vi "multi-mode-acquisition.vi"() -> ()   [LabVIEW 2014]
doc: "Acquires sequences from the Andor iXon camera. \"Multi-mode\" means that the VI can be configured to sequentially acquire frames in multiple modes with different light sources and numbers of frames in each mode. Each mode is collected into a separate aquisition directory. Acquisition can be time-lapsed with a settable delay interval between cycles; the selected laser(s) are shuttered whilst not acquiring. The ixon setup acquisition.vi front panel is displayed so that the user can set the acquisition parameters before acquiring."
uses:
  SubVIs/ctt's/Image size and binning.ctl
  SubVIs/ctt's/Camera Setup Acquisition.ctl
  SubVIs/ctt's/acquisition protocol multimode.ctl
  Shutter Control/Shutter SubVIs/ctts/laser shutters.ctl
  SubVIs/ctt's/Video acquisition state1.ctl
  <vilib>/vision/Image Controls.llb/IMAQ Image.ctl
  Shutter Control/Shutter SubVIs/ctts/user event shutter global.ctl
  SubVIs/Globals/Initilize Globals.vi
  File Directory/File-Locations-Global.vi
  TIRF Lock/autofocus-globals.vi
  Stage Control/stage-controller-globals.vi
panel:
  in  "Exposure Time (sec)":sgl(slide)=0.1 scale=0.001..10.0 scale format="%#_1g"
  in  "EM CCD Gain":u16(slide)=300 scale=0.01..300.0
  in  "Acquisition directory root path":path=path "c:/scratch"
  in  "Max Cycles":i32
  in  "Cycle Interval (s)":dbl format="%_2g"
  in  "Scan Fields":bool
  in  "Scan Field Options":T1(radio)
  in  "Max. number of acquisition files":i8(slide)=10 scale=0.0..50.0
  in  "Acquisition Protocol":T2
  in  "Quit":bool
  in  "Start":bool
  in  "Acquisition Parameters":T4={"Set Acquisition Mode"=enum."Single Scan", "Trigger Mode"=enum."Internal", "Set VS Speed"=1.0, "Pixel Rate"=enum."Standard CCD 3 Mhz 14 bits", "V Shift Amplitude"=enum."+1", "Readout Mode"=enum."Image", "Single Track \nSettings"={"centre"=0, "height"=1}, "Preamp Gain"=enum."1.0", "Number of\nAccumulations"=0, "Number of Kinetics"=1, "Accumulation\nCycle (s)"=1.0, "Kinetic Cycle Time (s)"=1.0, "High Capacity?"=FALSE} {"Single Track \nSettings"."centre" min=0 max=1024; "Single Track \nSettings"."height" min=1 max=1024; "Set VS Speed" min=0.0 format="%#_2f"}
  in  "Image Size":T5={"H Bin"=1.0, "V Bin"=1.0, "Left"=1.0, "Right"=1024.0, "Top"=1.0, "Bottom"=1024.0} {"V Bin" min=0.0; "H Bin" min=0.0 step=1.0}
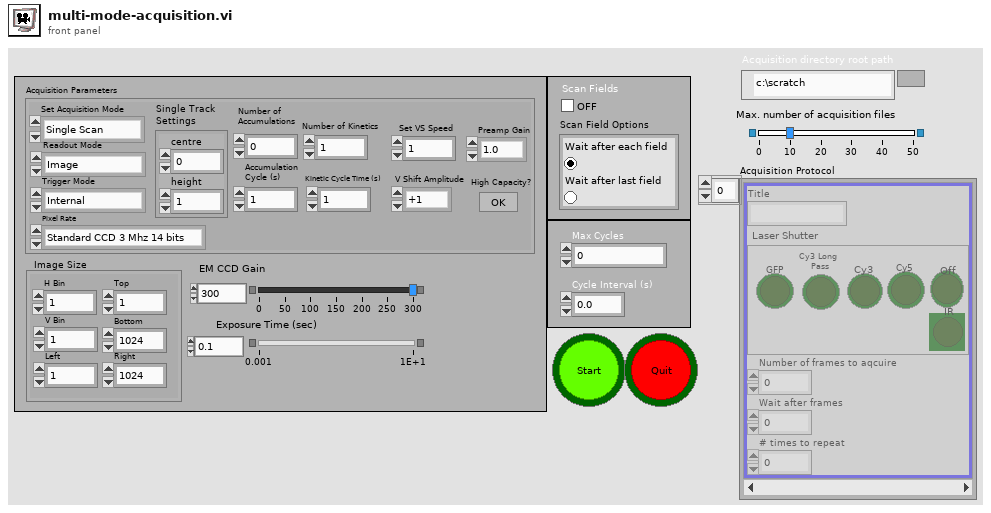
[diagram p1: front panel]
types:
  T1 = enum32{"Wait after each field", "Wait after last field"}
  T2 = typedef "acquisition protocol multimode.ctl" = cluster{"Title":string, "Laser Shutter":T3, "Number of frames to aqcuire":dbl, "Wait after frames":dbl, "# times to repeat":u32}[]
  T3 = typedef "laser shutters.ctl" = enum32{"No Selection", "GFP", "Cy3 Long \nPass", "Cy3", "Cy5", "Off", "IR"}
  T4 = typedef "Camera Setup Acquisition.ctl" = cluster{"Set Acquisition Mode":enum16{"(do nothing)", "Single Scan", "Accumulate", "Kinetics", "Fast Kinetics", "Run till abort"}, "Trigger Mode":enum16{"Internal", "External"}, "Set VS Speed":dbl, "Pixel Rate":enum16{"EM CCD 10 Mhz 14 bits", "EM CCD 5 Mhz 14 bits", "EM CCD 3 Mhz 14 bits", "EM CCD 1 Mhz 16 bits", "Standard CCD 3 Mhz 14 bits", "Standard CCD 1 Mhz 16 bits"}, "V Shift Amplitude":enum16{"normal", "+1", "+2", "+3", "+4"}, "Readout Mode":enum16{"Full Vertical Binning", "Multi-Track", "Random-Track", "Single-Track", "Image"}, "Single Track \nSettings":cluster{"centre":i32, "height":i32}, "Preamp Gain":enum16{"1.0", "2.4", "5.0"}, "Number of\nAccumulations":i32, "Number of Kinetics":i32, "Accumulation\nCycle (s)":dbl, "Kinetic Cycle Time (s)":dbl, "High Capacity?":bool}
  T5 = typedef "Image size and binning.ctl" = cluster{"H Bin":dbl, "V Bin":dbl, "Left":dbl, "Right":dbl, "Top":dbl, "Bottom":dbl}
  T6 = typedef "user event shutter global.ctl" = cluster{"Camera Shutter":bool, "Laser Shutter":enum32{"No Selection", "GFP", "Cy3 Long \nPass", "Cy3", "Cy5", "Off", "IR"}}
  T7 = enum32{"None", "Manual", "Auto - Image analysis", "Auto - Retro-reflection"}
  T8 = enum32{"No Selection", "GFP", "Cy3 Long \nPass", "Cy3", "Cy5", "Off", "IR"}
  T9 = cluster{"Title":string, "Laser Shutter":T3, "Number of frames to aqcuire":dbl, "Wait after frames":dbl, "# times to repeat":u32}
  T10 = cluster{"H Bin":dbl, "V Bin":dbl, "Left":dbl, "Right":dbl, "Top":dbl, "Bottom":dbl}
  T11 = cluster{"Frame Size (bytes)":i32, "Max Time (min)":i32, "Max Frames":i32, "Frames per acquisition file":i32, "Max time (s)":i32, "Max Space Req'd. (Gb)":dbl}
  T12 = typedef "Video acquisition state1.ctl" = cluster{"Pixel depth":enum32{"8 bits", "16 bits", "Float", "Complex", "RGB Chunky", "Compressed"}, "Width":dbl, "Height":dbl, "Buffer":T13, "Frames Acquired":u32, "Time of 1st frame":dbl, "TTB element zero":u32, "File Offsets Array":cluster{"offset":i32, "file number":u8}[], "TTB Array":u32[], "Sum Image (for averaging)":T13, "Time at end of last acquisition (ms)":u32, "Flow rate array":dbl[], "Temperature array":dbl[], "Field array":u16[], "Stage xyz array":dbl[][], "Current Filter Wheel Array":string[], "Laser Shutter Array":enum32{"No Selection", "GFP", "Cy3 Long \nPass", "Cy3", "Cy5", "Off", "IR"}[]}
  T13 = typedef "IMAQ Image.ctl" = refnum<image>
  T14 = typedef "Sequence file handle.ctl" = cluster{"Sequence files directory path":path, "Sequence files refnum array":refnum<file>[]}
  T15 = cluster{"Sequence files directory path":path, "Sequence files refnum array":refnum<file>[]}
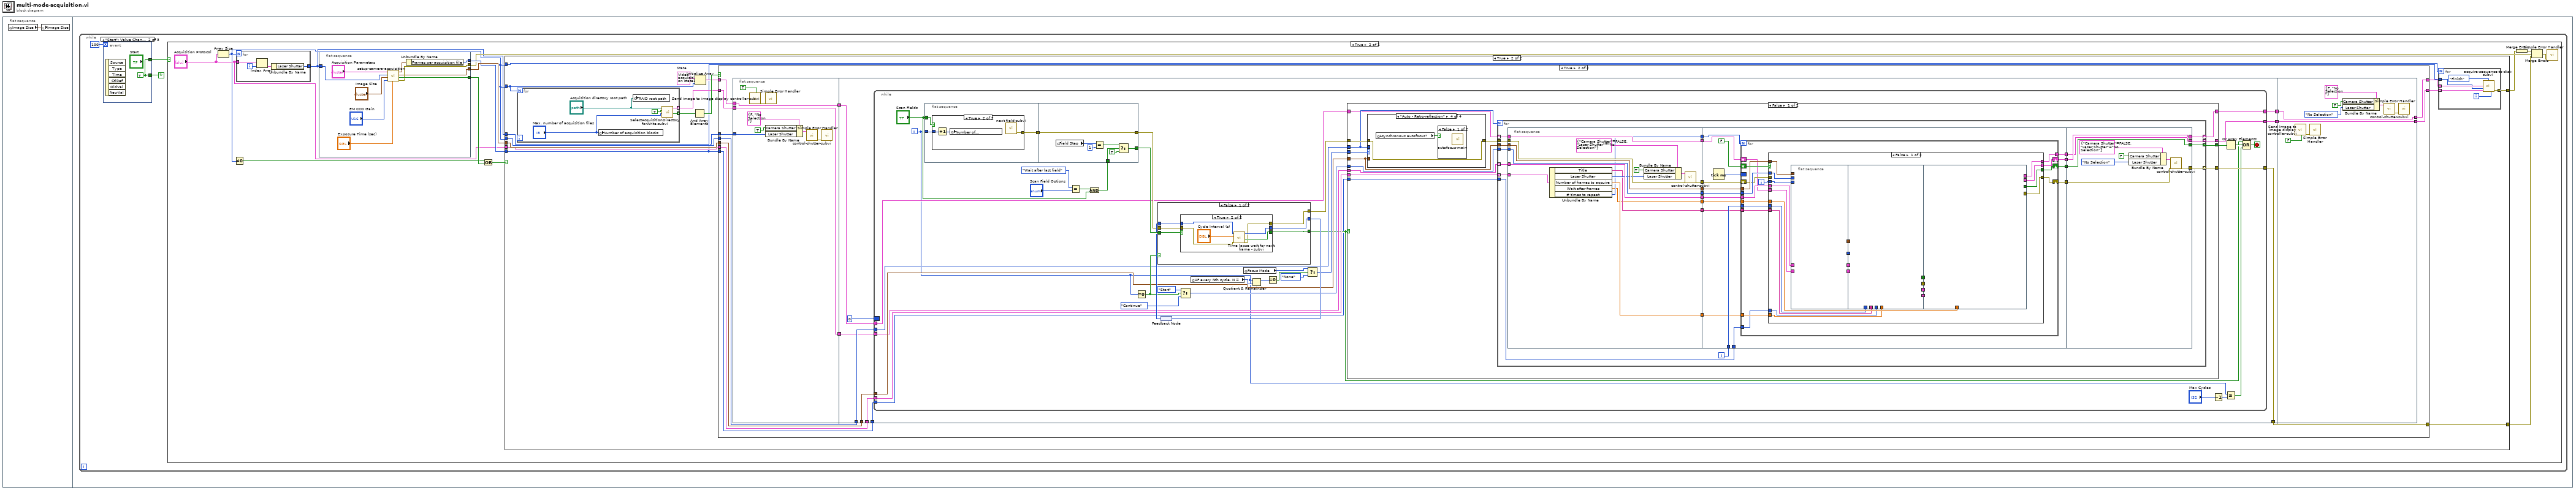
[diagram p0: block diagram]
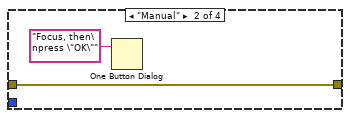
[diagram p7: hidden frame]
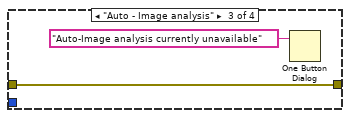
[diagram p8: hidden frame]
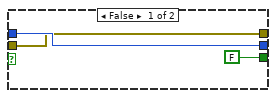
[diagram p11: hidden frame]
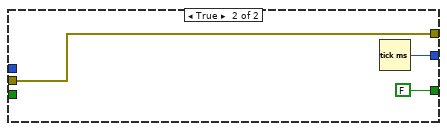
[diagram p12: hidden frame]
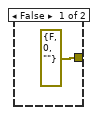
[diagram p13: hidden frame]
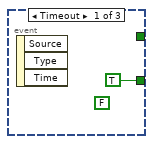
[diagram p14: hidden frame]
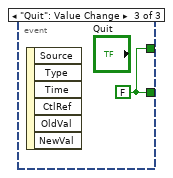
[diagram p15: hidden frame]
diagram:
  n1 = flat-sequence {
    frame #0 {
      n2 = global read "Initilize Globals.vi" "Image Size"() -> (w1:T5)
      n3 = local write "Image Size"(w1) -> ()
    }
    frame #1 {
      n4 = while {
        stop <- w3 continue-if-true
        n5 = event shown="[1] \"Start\": Value Change" {
          selector: _ -> [_ _ _]
          dyn-events: _ -> [_ _ _]
          timeout: 100 -> [_ _ _]
          tunnel: [TRUE w337 w338] -> w3
          tunnel: [_ w337 w338] -> w2
          event Timeout {
            (unwired) FALSE
            n6 = event-data() -> ()  [unwired: 1 in, 3 out]
          }
          event "Start": Value Change {
            w337 = TRUE
            n7 = event-data() -> ()  [unwired: 1 in, 6 out]
          }
          event "Quit": Value Change {
            w338 = FALSE
            n8 = event-data() -> ()  [unwired: 1 in, 6 out]
          }
        }
        n9 = case shown="True" w2 {
          frame False {
          }
          frame True {
            n10 = Array Size(array="Acquisition Protocol") -> (size(s)=w9:i32)
            n11 = Not Equal To 0?(x=w9) -> (x != 0?=w5:bool)
            n12 = for {
              N: w9 -> [_]
              tunnel: "Acquisition Protocol" -> [w21]
              tunnel: [w18] -> w6
              i -> [w20]
              n13 = Index Array(array=w21, index=w20) -> (element=w19:T9)
              n14 = Unbundle By Name(w19) -> ("Laser Shutter"=w18:T3)
            }
            n15 = flat-sequence {
              tunnel: [w331] -> w16
              tunnel: [w330] -> w11
              tunnel: [w328] -> w15
              tunnel: [w335] -> w12
              tunnel: w6 -> [w332]
              frame #0 {
                n16 = call "setup-camera-acquisition.vi"("Exposure Time (sec)"="Exposure Time (sec)", "EM CCD Gain"="EM CCD Gain", "Image Size"="Image Size", "Laser Shutter"=w332, "Acquisition Parameters"="Acquisition Parameters") -> ("Error Out"=w330:errorcluster, "Continue with \nacquisition?"=w331:bool, "Image Size Out"=w328:T10, "File properties"=w329:T11)  [unwired: 3 in]
                n17 = Unbundle By Name(w329) -> ("Frames per acquisition file"=w335:i32)
              }
            }
            n18 = Or(x=w5, y=w16) -> (x .or. y?=w17:bool)
            n19 = case shown="True" w17 {
              tunnel: w9 -> [_ w37]
              tunnel: w15 -> [_ w33]
              tunnel: "Acquisition Protocol" -> [_ w32]
              tunnel: w9 -> [_ w31]
              tunnel: [_ w30] -> w14
              tunnel: w9 -> [_ w29]
              tunnel: w12 -> [_ w23]
              tunnel: [_ w26] -> w7
              tunnel: w6 -> [_ w22]
              frame False {
              }
              frame True {
                w36 = T12 {"Pixel depth"=enum."8 bits", "Width"=0.0, "Height"=0.0, "Buffer"=refnum, "Frames Acquired"=0, "Time of 1st frame"=0.0, "TTB element zero"=0, "File Offsets Array"=[], "TTB Array"=[], "Sum Image (for averaging)"=refnum, "Time at end of last acquisition (ms)"=0, "Flow rate array"=[], "Temperature array"=[], "Field array"=[], "Stage xyz array"=[], "Current Filter Wheel Array"=[], "Laser Shutter Array"=[]}  # State
                n20 = for {
                  N: w37 -> [_]
                  tunnel: [w323] -> w35 mode=indexing
                  tunnel: [w322] -> w28 mode=indexing
                  n21 = global write "Initilize Globals.vi" "Number of acquisition blocks"("Max. number of acquisition files") -> ()
                  n22 = global write "File-Locations-Global.vi" "RAID root path"("Acquisition directory root path") -> ()
                  n23 = call "SelectAcquisitionDirectoryforWrite-subvi.vi"("Number of acquisition files"="Max. number of acquisition files", "Autostart?"=TRUE, "Acquisition directory root path"="Acquisition directory root path") -> ("OK?"=w323:bool, "Sequence files handle"=w322:T14)  [unwired: 7 in]
                }
                n24 = And Array Elements(Boolean array=w35) -> (logical AND=w34:bool)
                n25 = Initialize Array(w36, w37) -> (w27:T12[])
                n26 = case shown="True" w34 {
                  tunnel: w33 -> [_ w59]
                  tunnel: w32 -> [_ w58]
                  tunnel: w31 -> [_ w57]
                  tunnel: [_ w56] -> w30
                  tunnel: w28 -> [w45 w54]
                  tunnel: w27 -> [w44 w48]
                  tunnel: w23 -> [_ w53]
                  tunnel: [w44 w51] -> w25
                  tunnel: [w45 w49] -> w24
                  tunnel: w22 -> [_ w46]
                  frame False {
                  }
                  frame True {
                    n27 = flat-sequence {
                      tunnel: [w62] -> w55
                      tunnel: w54 -> [w62]
                      tunnel: w48 -> [w61]
                      tunnel: [w61] -> w47
                      tunnel: w46 -> [w60]
                      tunnel: w59 -> [w77]
                      tunnel: w58 -> [w76]
                      tunnel: w57 -> [w75]
                      tunnel: [w74] -> w56
                      tunnel: w55 -> [w73]
                      tunnel: w53 -> [w72]
                      tunnel: [w71] -> w52
                      tunnel: [w70] -> w50
                      tunnel: w47 -> [w69]
                      tunnel: w52 -> [w313]
                      tunnel: [w313] -> w51
                      tunnel: w50 -> [w312]
                      tunnel: [w312] -> w49
                      frame #0 {
                        n28 = call "Send image to image display controller-subvi.vi"("Start display controller?"=TRUE) -> ("error out"=w64:errorcluster)  [unwired: 8 in, 1 out]
                        n29 = call <vilib>:"Simple Error Handler.vi"("error in (no error)"=w64) -> ()  [unwired: 1 in, 8 out]
                        n30 = Bundle By Name(cluster=T6 {"Camera Shutter"=FALSE, "Laser Shutter"=enum."No Selection"} ("Shutter Control"), "Camera Shutter"=TRUE, "Laser Shutter"=w60) -> (w66:T6)
                        n31 = call "control-shutter-subvi.vi"("Shutter Control"=w66) -> ("Error Out"=w65:errorcluster)  [unwired: 10 in]
                        n32 = call <vilib>:"Simple Error Handler.vi"("error in (no error)"=w65) -> ()  [unwired: 1 in, 8 out]
                      }
                      frame #1 {
                        n33 = while {
                          border: 0 -> [_]
                          tunnel: w77 -> [w98]
                          tunnel: w76 -> [w95]
                          tunnel: w75 -> [w94]
                          tunnel: [w91] -> w74
                          tunnel: w73 -> [w89]
                          tunnel: w69 -> [w86]
                          tunnel: w72 -> [w85]
                          tunnel: [w84] -> w71
                          tunnel: [w83] -> w70
                          i -> [w79]
                          stop <- w92 stop-if-true
                          n34 = flat-sequence {
                            tunnel: "Scan Fields" -> [w300]
                            tunnel: [w299] -> w112
                            tunnel: w79 -> [w298]
                            tunnel: w113 -> [w310]
                            tunnel: w112 -> [w309]
                            tunnel: [w309] -> w97
                            tunnel: [w308] -> w111
                            frame #0 {
                              n35 = case shown="True" w300 {
                                tunnel: [errorcluster {"status"=FALSE, "code"=0, "source"=""} ("Error Out") w304] -> w299
                                tunnel: w298 -> [_ w303]
                                frame False {
                                }
                                frame True {
                                n36 = Increment(x=w303) -> (x+1=w302:i32)
                                n37 = global write "stage-controller-globals.vi" "Number of \nField Steps"(w302) -> ()
                                n38 = call "next field-subvi.vi"() -> ("Error Out"=w304:errorcluster)  [unwired: 11 in]
                                }
                              }
                            }
                            frame #1 {
                              n39 = global read "stage-controller-globals.vi" "Field Step"() -> (w305:u32)
                              n40 = Equal?(x=w305, y=u32 1) -> (x = y?=w307:bool)
                              n41 = Select(t=w307, s=w310, f=TRUE) -> (s? t:f=w308:bool)
                            }
                          }
                          n42 = Equal?(x=T1."Wait after last field" ("y"), y="Scan Field Options") -> (x = y?=w116:bool)
                          n43 = And(x=w116, y="Scan Fields") -> (x .and. y?=w113:bool)
                          n44 = Equal To 0?(x=w79) -> (x = 0?=w108:bool)
                          n45 = feedback #1() -> (w109:u32)
                          n46 = case shown="False" w108 {
                            tunnel: w111 -> [w285 _]
                            tunnel: [w283 w297] -> w110
                            tunnel: w109 -> [w282 _]
                            tunnel: [w284 FALSE] -> w87
                            tunnel: w97 -> [w281 w295]
                            tunnel: [w280 w295] -> w96
                            frame False {
                              n47 = case shown="True" w285 {
                                tunnel: [FALSE w291] -> w284
                                tunnel: [w287 w293] -> w283
                                tunnel: w282 -> [w287 w294]
                                tunnel: w281 -> [w286 w290]
                                tunnel: [w286 w289] -> w280
                                frame False {
                                }
                                frame True {
                                n48 = call "Time lapse wait for next frame - subvi.vi"("Error In"=w290, "Frame Interval (s)"="Cycle Interval (s)", "Time of last frame in"=w294) -> ("Error Out"=w289:errorcluster, "Stopped?"=w291:bool, "Time of this frame out (ms)"=w293:i32)  [unwired: 5 in, 1 out]
                                }
                              }
                            }
                            frame True {
                              n49 = Tick Count (ms)() -> (millisecond timer value=w297:u32)
                            }
                          }
                          n50 = feedback-in #1(w110) -> ()
                          n51 = Select(t=enum16{"Start", "Continue", "Finish"}."Start" ("Operation"), s=w108, f=enum16{"Start", "Continue", "Finish"}."Continue" ("Operation")) -> (s? t:f=w102:enum16{"Start", "Continue", "Finish"})
                          n52 = global read "autofocus-globals.vi" "AF every Nth cycle, N ="() -> (w105:u32)
                          n53 = global read "autofocus-globals.vi" "Focus Mode"() -> (w103:T7)
                          n54 = Quotient & Remainder(x=w79, y=w105) -> (x-y*floor(x/y)=w107:u32)  [unwired: 1 out]
                          n55 = Equal To 0?(x=w107) -> (x = 0?=w106:bool)
                          n56 = Select(t=w103, s=w106, f=T7."None") -> (s? t:f=w101:T7)
                          n57 = case shown="False" w87 {
                            tunnel: w102 -> [w123 _]
                            tunnel: w101 -> [w130 _]
                            tunnel: w98 -> [w122 _]
                            tunnel: w96 -> [w129 _]
                            tunnel: w95 -> [w128 _]
                            tunnel: w94 -> [w127 _]
                            tunnel: [w126 _] -> w91
                            tunnel: [w125 _] -> w90
                            tunnel: w89 -> [w124 w279]
                            tunnel: w86 -> [w121 w278]
                            tunnel: w85 -> [w120 _]
                            tunnel: [w118 w278] -> w84
                            tunnel: [w117 w279] -> w83
                            frame False {
                              n58 = case shown="\"Auto - Retro-reflection\"" w130 {
                                tunnel: w122 -> [_ _ _ _]
                                tunnel: w129 -> [w271 w272 w275 w276]
                                tunnel: [w271 w272 w275 w276] -> w119
                                tunnel: w127 -> [_ _ _ _]
                                frame "None", Default {
                                }
                                frame "Manual" {
                                n59 = One Button Dialog(message="Focus, then\npress \"OK\"") -> ()  [unwired: 2 out]
                                }
                                frame "Auto - Image analysis" {
                                n60 = One Button Dialog(message="Auto-Image analysis currently unavailable") -> ()  [unwired: 2 out]
                                }
                                frame "Auto - Retro-reflection" {
                                n61 = global read "autofocus-globals.vi" "Asynchronous autofocus?"() -> (w277:bool)
                                n62 = case shown="False" w277 {
                                frame False {
                                n63 = call "autofocus-main.vi"() -> ()  [unwired: 12 in]
                                }
                                frame True {
                                }
                                }
                                }
                              }
                              n64 = for {
                                N: w127 -> [_]
                                tunnel: w128 -> [w140] mode=indexing
                                tunnel: [w131] -> w126 mode=indexing
                                tunnel: [w155] -> w125 mode=indexing
                                tunnel: w124 -> [w154] mode=indexing
                                tunnel: w123 -> [w153]
                                tunnel: w122 -> [w152]
                                tunnel: w121 -> [w146] mode=indexing
                                tunnel: w120 -> [w150]
                                tunnel: w119 -> [w149]
                                tunnel: [w148] -> w118 mode=indexing
                                tunnel: [w147] -> w117 mode=indexing
                                i -> [w151]
                                n65 = flat-sequence {
                                tunnel: w146 -> [w167]
                                tunnel: w149 -> [w165]
                                tunnel: w152 -> [w168]
                                tunnel: w153 -> [w169]
                                tunnel: w154 -> [w170]
                                tunnel: [w170] -> w145
                                tunnel: [w169] -> w144
                                tunnel: [w168] -> w143
                                tunnel: [w164] -> w142
                                tunnel: [w167] -> w141
                                tunnel: w140 -> [w166]
                                tunnel: [w159] -> w139
                                tunnel: [w158] -> w138
                                tunnel: [w157] -> w137
                                tunnel: [w156] -> w136
                                tunnel: w151 -> [w182]
                                tunnel: w150 -> [w181]
                                tunnel: w145 -> [w185]
                                tunnel: w144 -> [w184]
                                tunnel: w143 -> [w183]
                                tunnel: w142 -> [w180]
                                tunnel: w141 -> [w176]
                                tunnel: w139 -> [w175]
                                tunnel: w138 -> [w174]
                                tunnel: w137 -> [w173]
                                tunnel: w136 -> [w172]
                                tunnel: [w187] -> w135
                                tunnel: [w179] -> w134
                                tunnel: [w178] -> w133
                                tunnel: [w171] -> w132
                                tunnel: [w268] -> w147
                                tunnel: [w269] -> w148
                                tunnel: [w270] -> w155
                                tunnel: w135 -> [w270]
                                tunnel: w134 -> [w269]
                                tunnel: w133 -> [w268]
                                tunnel: w132 -> [w267]
                                tunnel: [w266] -> w131
                                frame #0 {
                                n66 = Unbundle By Name(w166) -> ("Title"=w159:string, "Laser Shutter"=w160:T3, "Number of frames to aqcuire"=w158:dbl, "Wait after frames"=w156:dbl, "# times to repeat"=w157:u32)
                                n67 = Bundle By Name(cluster=T6 {"Camera Shutter"=FALSE, "Laser Shutter"=enum."No Selection"} ("Shutter Control"), "Camera Shutter"=TRUE, "Laser Shutter"=w160) -> (w162:T6)
                                n68 = call "control-shutter-subvi.vi"("Error In"=w165, "Shutter Control"=w162) -> ("Error Out"=w164:errorcluster)  [unwired: 9 in]
                                }
                                frame #1 {
                                n69 = Tick Count (ms)() -> (millisecond timer value=w177:u32)
                                n70 = for {
                                N: w173 -> [_]
                                shift-right: [w203] -> w171
                                shift-left: w180 -> [w191]
                                shift-right: [w202] -> w187
                                shift-left: FALSE -> [w201]
                                tunnel: w172 -> [w200]
                                tunnel: w185 -> [w199]
                                tunnel: w175 -> [w198]
                                tunnel: w174 -> [w197]
                                tunnel: w184 -> [w196]
                                tunnel: w183 -> [w195]
                                tunnel: w182 -> [w193]
                                tunnel: w181 -> [w192]
                                tunnel: [w189] -> w178
                                border: w177 -> [_]
                                shift-right: [w190] -> w179
                                shift-left: w176 -> [w188]
                                i -> [w194]
                                n71 = case shown="False" w201 {
                                selector: w201 -> [_ w260]
                                tunnel: [w225 w261] -> w203
                                tunnel: [w224 w260] -> w202
                                tunnel: w200 -> [w223 _]
                                tunnel: w199 -> [w222 w258]
                                tunnel: w198 -> [w220 _]
                                tunnel: w197 -> [w219 _]
                                tunnel: w196 -> [w218 _]
                                tunnel: w195 -> [w217 _]
                                tunnel: w194 -> [w215 _]
                                tunnel: w193 -> [w213 _]
                                tunnel: w188 -> [w211 w259]
                                tunnel: w192 -> [w210 _]
                                tunnel: w191 -> [_ w261]
                                tunnel: [w209 w259] -> w190
                                tunnel: [w208 w258] -> w189
                                frame False {
                                n72 = flat-sequence {
                                tunnel: w222 -> [w233]
                                tunnel: [w233] -> w221
                                tunnel: w218 -> [w231]
                                tunnel: w217 -> [w232]
                                tunnel: [w232] -> w216
                                tunnel: w215 -> [w229]
                                tunnel: [w227] -> w214
                                tunnel: [w226] -> w212
                                tunnel: w211 -> [w226]
                                tunnel: w221 -> [w246]
                                tunnel: w220 -> [w236]
                                tunnel: w219 -> [w239]
                                tunnel: w216 -> [w245]
                                tunnel: w214 -> [w235]
                                tunnel: w213 -> [w243]
                                tunnel: w212 -> [w244]
                                tunnel: w210 -> [w242]
                                tunnel: [w240] -> w207
                                tunnel: [w238] -> w206
                                tunnel: [w237] -> w205
                                tunnel: [w234] -> w204
                                tunnel: [w255] -> w225
                                tunnel: [w253] -> w224
                                tunnel: w223 -> [w252]
                                tunnel: w206 -> [w250]
                                tunnel: w207 -> [w249]
                                tunnel: [w249] -> w209
                                tunnel: [w248] -> w208
                                tunnel: w205 -> [w248]
                                tunnel: w204 -> [w247]
                                frame #0 {
                                n73 = Equal To 0?(x=w229) -> (x = 0?=w230:bool)
                                n74 = Select(t=w231, s=w230, f=enum16{"Start", "Continue", "Finish"}."Continue" ("Operation")) -> (s? t:f=w227:enum16{"Start", "Continue", "Finish"})
                                }
                                frame #1 {
                                n75 = call "acquire-sequence-to-disk-subvi.vi"("Image Size"=w245, "Operation"=w235, "Number of frames to acquire"=w239, "State In"=w244, "Frames per acquisition file"=w242, "Sequence files handle"=w246, "Pressing stop \nautomatically runs finish?"=FALSE ("Pressing stop automatically runs finish?"), "Display Window Title"=w236, "Display Window Number"=w243) -> ("Done?"=w238:bool, "State Out"=w240:T12, "Sequence files handle out"=w237:T15, "Error Out"=w234:errorcluster)  [unwired: 3 in]
                                }
                                frame #2 {
                                n76 = feedback #2() -> (w256:u32)
                                n77 = call "Time lapse wait for next frame - subvi.vi"("Error In"=w247, "Frame Interval (s)"=w252, "Time of last frame in"=w256) -> ("Error Out"=w255:errorcluster, "Stopped?"=w251:bool, "Time of this frame out (ms)"=w257:i32)  [unwired: 5 in, 1 out]
                                n78 = feedback-in #2(w257) -> ()
                                n79 = Unbundle By Name(w255) -> ("status"=w254:bool)
                                n80 = Compound Arithmetic op=OR(w250, w251, w254) -> (w253:bool)
                                }
                                }
                                }
                                frame True {
                                }
                                }
                                }
                                }
                                frame #2 {
                                n81 = Bundle By Name(cluster=T6 {"Camera Shutter"=FALSE, "Laser Shutter"=enum."No Selection"} ("Shutter Control"), "Camera Shutter"=FALSE, "Laser Shutter"=T8."No Selection") -> (w264:T6)
                                n82 = call "control-shutter-subvi.vi"("Error In"=w267, "Shutter Control"=w264) -> ("Error Out"=w266:errorcluster)  [unwired: 9 in]
                                }
                                }
                              }
                            }
                            frame True {
                            }
                          }
                          n83 = Decrement(x="Max Cycles") -> (x-1=w80:i32)
                          n84 = Or Array Elements(Boolean array=w90) -> (logical OR=w93:bool)
                          n85 = Greater Or Equal?(x=w79, y=w80) -> (x >= y?=w88:bool)
                          n86 = Compound Arithmetic op=OR(w87, w93, w88) -> (w92:bool)
                        }
                      }
                      frame #2 {
                        n87 = call "Send image to image display controller-subvi.vi"("Quit display controller?"=FALSE) -> ("error out"=w316:errorcluster)  [unwired: 8 in, 1 out]
                        n88 = call <vilib>:"Simple Error Handler.vi"("error in (no error)"=w316) -> ()  [unwired: 1 in, 8 out]
                        n89 = Bundle By Name(cluster=T6 {"Camera Shutter"=FALSE, "Laser Shutter"=enum."No Selection"} ("Shutter Control"), "Camera Shutter"=FALSE, "Laser Shutter"=T8."No Selection") -> (w318:T6)
                        n90 = call "control-shutter-subvi.vi"("Shutter Control"=w318) -> ("Error Out"=w317:errorcluster)  [unwired: 10 in]
                        n91 = call <vilib>:"Simple Error Handler.vi"("error in (no error)"=w317) -> ()  [unwired: 1 in, 8 out]
                      }
                    }
                  }
                }
                n92 = for {
                  N: w29 -> [_]
                  tunnel: [w43] -> w26 mode=indexing
                  tunnel: w25 -> [w41] mode=indexing
                  tunnel: w24 -> [w42] mode=indexing
                  tunnel: w23 -> [w38]
                  i -> [w40]
                  n93 = call "acquire-sequence-to-disk-subvi.vi"("Operation"=enum16{"Start", "Continue", "Finish"}."Finish", "State In"=w41, "Frames per acquisition file"=w38, "Sequence files handle"=w42, "Display Window Number"=w40) -> ("Error Out"=w43:errorcluster)  [unwired: 7 in, 3 out]
                }
              }
            }
            n94 = Merge Errors(w7) -> (w8:errorcluster)
            n95 = Merge Errors(w8, w11, w14) -> (w13:errorcluster)
            n96 = call <vilib>:"Simple Error Handler.vi"("error in (no error)"=w13) -> ()  [unwired: 4 in, 5 out]
          }
        }
      }
    }
  }
